vi "CASE Experiment Refinement.vi"() -> ()   [LabVIEW 2014]
uses:
  <vilib>/Simulation/Scripting/Companion Diagram/SimConfigNode/SimParams.ctl
  <vilib>/Simulation/Scripting/Companion Diagram/SimConfigNode/_simSolvers.ctl
  <vilib>/Simulation/Implementation/Shared/SIMSCR Execution Mode.ctl
  <vilib>/Platform/TimedLoop/XDataNode/timing_clust.ctl
  <vilib>/Platform/TimedLoop/XDataNode/nitl_modes.ctl
  <vilib>/Platform/TimedLoop/XDataNode/wakeup.ctl
  <vilib>/Simulation/Param Hierarchy/Typedefs/SIMPH Param Control Actions.ctl
  <vilib>/addons/control/pid/pid.llb/PID Structure.ctl
  <vilib>/addons/control/pid/pid.llb/PID Gain Unit.ctl
  <vilib>/Simulation/Implementation/Shared/NILVSim_ParamChanged.vi
  <vilib>/Simulation/Implementation/Shared/NILVSim_FinishedLate.vi
  <vilib>/Simulation/Implementation/Shared/NILVSIM_BeginStep.vi
  <vilib>/Simulation/ContinuousLinear/Implementation/NILVSim Transfer Function.llb/SIM Transfer Function Distributor (SISO).vi
  <vilib>/Simulation/ContinuousLinear/Implementation/NILVSim Transport Delay.llb/SIM Transport Delay Direct (scalar).vi
  <vilib>/Simulation/ContinuousLinear/Implementation/NILVSim Transfer Function.llb/SIM Transfer Function Collector (SISO).vi
  <vilib>/Simulation/SignalDisplay/Implementation/NILVSim Time Waveform.llb/SIM Time Waveform (vector).vi
  <vilib>/Simulation/Implementation/Shared/NILVSim_Manager.vi
  <vilib>/Utility/error.llb/Clear Errors.vi
  <vilib>/Simulation/Implementation/Shared/NILVSim_FinalizeModel.vi
  <vilib>/FPGAPlugInAG/myRIO-1900/niLvFpga_Open_myRIO-1900.vi
  <vilib>/rvi/interface/common/dynamic/niFpgaDynamicAddResources.vi
  <vilib>/Utility/error.llb/Error Cluster From Error Code.vi
  <vilib>/rvi/errors/niLvFpgaAdjustHostInterfaceError.vi
  <vilib>/Utility/file.llb/Write To Spreadsheet File (DBL).vi
  <vilib>/FPGAPlugInAG/Dynamic/niLvFpga_Close_Dynamic.vi
  <vilib>/Simulation/Implementation/Shared/SIM Unbundle Sim Info.vi
  <vilib>/Simulation/Implementation/Shared/SIMSH Read Queue.vi
  <vilib>/Simulation/Implementation/Shared/NILVSim_Initialize.vi
  <vilib>/addons/control/pid/pid.llb/PID Structure Conversion.vi
  <vilib>/addons/control/pid/pid.llb/PID Structure Conversion (DBL).vi
  <vilib>/addons/control/pid/pid.llb/PID Lead-Lag.vi
  <vilib>/addons/control/pid/pid.llb/PID Lead-Lag (DBL).vi
  <vilib>/addons/control/pid/pid.llb/PID Advanced.vi
  <vilib>/addons/control/pid/pid.llb/PID Advanced (DBL).vi
  <vilib>/Simulation/Utility/Implementation/NILVSim Get Time and IsAcceptedStep.vi
  <vilib>/Simulation/Implementation/Shared/NILVSim_GetModelError.vi
  <vilib>/Simulation/Implementation/Shared/SIM Bundle Sim Info.vi
  <vilib>/addons/Control Design/_Model Construction/Special Model Creation.llb/Special Model Creation SubVI/CD Create Pade Delay Model.vi
  <vilib>/addons/Control Design/_Model Construction/Special Model Creation.llb/Special Model Creation SubVI/CD Create 2nd Order Model.vi
  <vilib>/rvi/interface/nirviOpenFPGA/nirviOpenFPGA.xnode
  FPGA Bitfiles/Test_FPGATarget_CurrentControl_60eBuCSPTsI.lvbitx
  Current Control.vi
  <vilib>/rvi/interface/nirviReadWriteControl/nirviReadWriteControl.xnode
  <vilib>/rvi/interface/nirviCloseFPGA/nirviCloseFPGA.xnode
  <vilib>/Simulation/Scripting/Companion Diagram/SimConfigNode/SimDog.xnode
  <vilib>/Platform/TimedLoop/XDataNode/XDataNode.xnode
  <vilib>/Simulation/Implementation/XNodeFramework/SimXNode/SimX.xnode
  <vilib>/rvi/interface/Simulation/niFpgaSimulationCallBeginRW.vi
  <vilib>/addons/Control Design/_Model Construction/NI_LinSys_Model Creation.lvlib
  <vilib>/addons/Control Design/_Model Construction/Model Creation.llb/Model Creation SubVI/cd_Create Zero-Pole-Gain Model.vi
  <vilib>/addons/Control Design/_Model Conversions/NI_CD_Model Type.lvlib
  <vilib>/addons/Control Design/_Model Conversions/Model Type.llb/Model Conversion SubVI/cd_Convert Zero-Pole-Gain to Transfer Function Model.vi
  <vilib>/addons/Control Design/_Model Delay/NI_CD_Model Delay.lvlib
  <vilib>/addons/Control Design/_Model Delay/Model Delay.llb/Model Delay subVIs/cd_Convert Delay with Pade Approx (TF).vi
  <vilib>/addons/Control Design/_Model Interconnection/NI_CD_Model Interconnection.lvlib
  <vilib>/addons/Control Design/_Model Interconnection/Model Interconnection.llb/Model Interconnection SubVI/cd_Series (TF and TF).vi
  <vilib>/addons/control/pid/NI_PID_pid.lvlib
  <vilib>/addons/Control Design/_Model Construction/NI_CD_Special Model Creation.lvlib
  <vilib>/Simulation/ContinuousLinear/Implementation/NILVSim Transfer Function.llb/SIM Transfer Function (SISO).vi
  <vilib>/Utility/file.llb/Write To Spreadsheet File (I64).vi
  NiFpgaLv.dll
  <vilib>/Platform/TimedLoop/XDataNode/XDNodeRunTimeDep.lvlib
  <vilib>/Simulation/Implementation/Shared/NI_SIM_Implementation.lvlib
panel:
  out "PV1:":dbl(slide)=50.762476114859936 scale=0.0..100.0
  in  "ControlTab":enum32{"PID Parameters", "PI Parameters"}(tab)
  in  "PID BETA":dbl(slide)=1.0 scale=0.0..1.0
  in  "Gamma PID":dbl(slide) scale=0.0..1.0
  in  "Manual Mode PID":dbl(slide) scale=0.0..50.0
  in  "auto? (T)":bool=TRUE
  in  "reinitialize? (F)":bool
  in  "Linearity PID":dbl(slide)=1.0 scale=0.0..1.0
  in  "Alpha PID":dbl(slide)=nan scale=0.0..1.0
  in  "Feedforward\nLag Time (min)":dbl(slide)=0.9102981779915218 scale=0.01..10.0
  in  "auto? (T) PI":bool=TRUE
  in  "PI beta":dbl(slide)=1.0 scale=0.0..1.0
  in  "reinitialize? PI":bool
  in  "Linearity PI":dbl(slide)=1.0 scale=0.0..1.0
  in  "Alpha PI":dbl(slide)=nan scale=0.0..1.0
  in  "Gamma PI":dbl(slide)=nan scale=0.0..1.0
  in  "Manual Mode PI":dbl(slide) scale=0.0..50.0
  out "PI Gains":T1
  out "PD Gains":T1
  out "Error":errorcluster
  in  "?":enum32{"RT Response", "Excitation/Response"}(tab)
  in  "SP1:":dbl(slide)=40.87020302841148 min=0.0 max=0.0 scale=20.0..27.45
  out "MV1:":dbl(slide)=100.0 scale=-100.0..100.0
  out "SP2:":dbl(slide)=140.87020302841148 min=0.0 max=0.0 scale=0.0..100.0
  out "control valve":dbl=86.66603993277398 format="%.2f"
  out "Kinect Measurement vs. IAB Height":waveform(dbl)[](graph)
  out "Ref Head Pose":dbl(slide)=50.762476114859936 scale=20.0..27.0
  out "Bladder\nHeight":dbl(slide)=49.279730305904245 scale=0.0..100.0 scale format="%.2f"
  out "Process Chart":cluster{"SP1:":dbl, "output":dbl, "output":dbl}(graph)
  in  "stop":bool
  out "Status?":bool
  # "Instructions\n\nThis is a cascade PID and PI feedforward surge bladder controller\n\n1. Make sure the GAMMA value for the PID is set to 1 so as to apply the  max weight to the error value of the derivative kick action\n2. Make GAMMA for PI control action equal to 0 since we are not weighting the derivative kick here\n3. Linearity value should be 1 for both  controllers to avoid parabolic response. 1 makes your response linear.\n4. Alpha is the derivative filter time constant. To make the PID in feedforward critically damped, use a value of 1 here. Make Alpha for PI 0.\n5.  Beta is the value of the relative emphasis of disturbance rejection to setpoint tracking. Make Beta 1; else make beta between 0 and 1 to accommodate disturbances such as load changes\n\nCopyright June 2015. Olalekan P. Ogunmolu"
  # "Gamma specifies an amount by which to weight the error applied to derivative action. The default value is 0, which avoids the derivative kick, or sudden change in controller output, that can occur after a change in the setpoint value. Since this is a cascade PID, derivative kick is not a concern, increasing gamma might improve the speed of the first PID controller.\n\nBeta specifies the relative emphasis of disturbance rejection to setpoint tracking. The default value of 1 is appropriate for most applications. You can use a smaller value between 0 and 1 to specify emphasis on disturbance rejection, such as process load changes. This VI resizes the beta input array to match the size of the process variable input array. \n\nManual control specifies the value of the control output when auto? is FALSE. This VI resizes the manual control input array to match the size of the process variable input array. \n\nLinearity specifies the linearity of the error response. The valid range for linearity is 0 to 1. A value of 1 provides a normal linear response, while a value of 0.1 provides an approximately parabolic response. The VI uses this value in the nonlinear error calculation and the nonlinear gain factor calculation. \n\nAlpha specifies the derivative filter time constant. Increasing this value increases damping of derivative action. alpha can be a value between 0 and 1 or NaN, which specifies that no derivative filter is applied. \n\nAuto? specifies whether to use automatic or manual control. In some situations, you might need to switch off the PID controller and operate the system in manual, or open-loop, mode. The default is TRUE. When auto? is TRUE, this VI uses automatic control. When auto? is FALSE, this VI uses manual control. This VI uses bumpless transfer from manual control to automatic control."
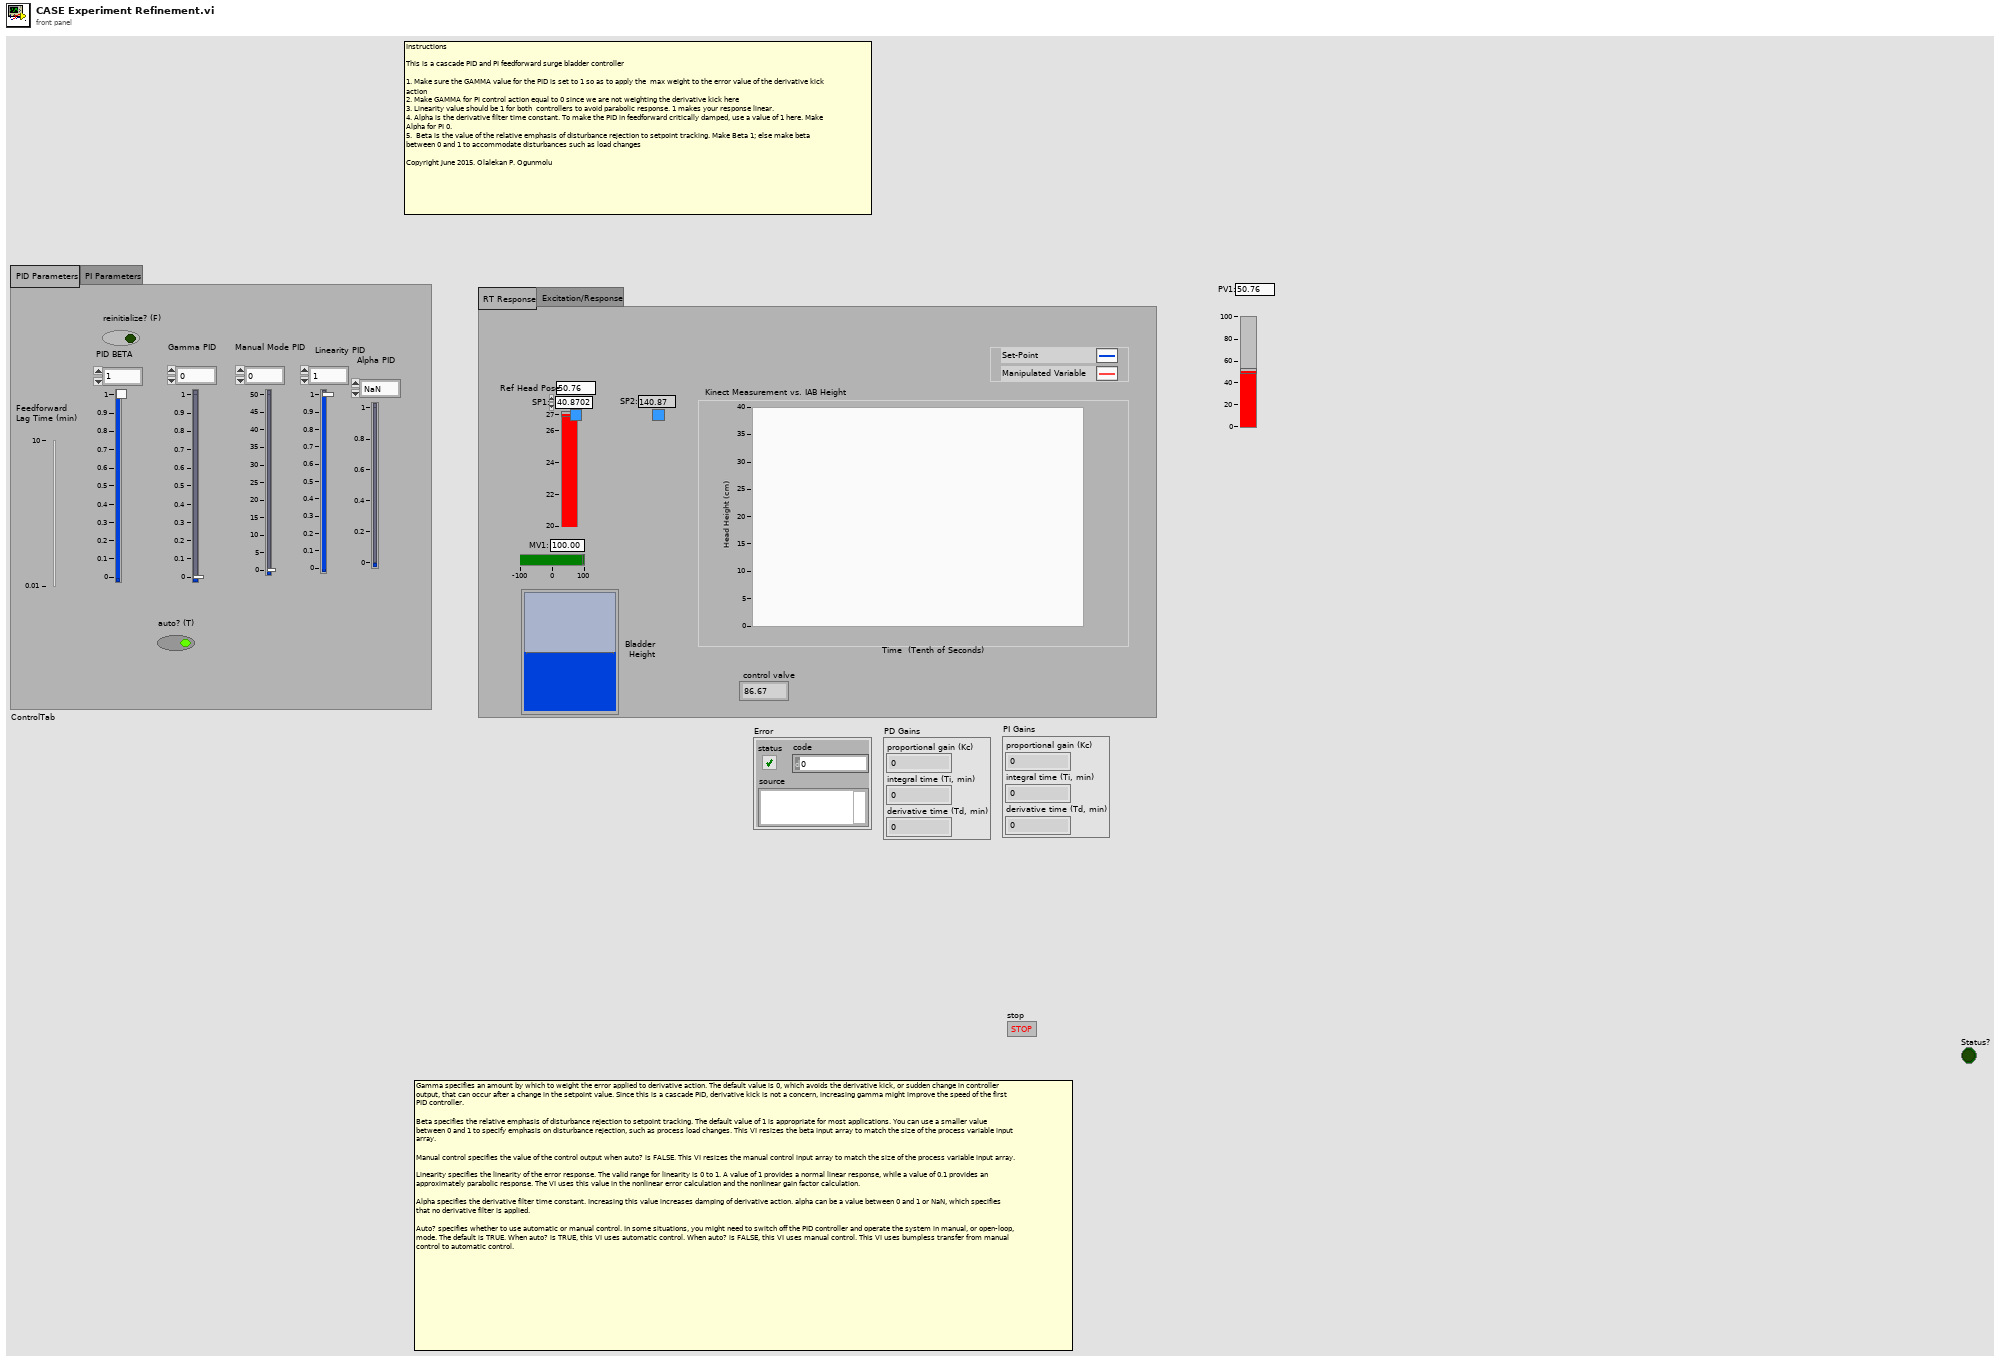
[diagram p1: front panel]
types:
  T1 = cluster{"proportional gain (Kc)":dbl, "integral time (Ti, min)":dbl, "derivative time (Td, min)":dbl}
  T2 = enum16{"big-endian, network order", "native, host order", "little-endian"}
  T3 = typedef "NI_LinSys_Model Typedefs.lvlib/CD Zero-Pole-Gain Model (MIMO).ctl" = cluster{"properties":T4, "zero-pole-gain(s)":T5[][]}
  T4 = typedef "NI_LinSys_Model Typedefs.lvlib/CD General Elements.ctl" = cluster{"Model name":string, "Input names":string[], "Output names":string[], "Input Delays":dbl[], "Output Delays":dbl[], "Sampling Time":dbl, "Notes":string}
  T5 = typedef "NI_LinSys_Model Typedefs.lvlib/CD Zero-Pole-Gain Model (SISO).ctl" = cluster{"Gain":dbl, "Zeros":cdb[], "Poles":cdb[], "delay":dbl}
  T6 = typedef "NI_LinSys_Model Typedefs.lvlib/CD Transfer Function Model (MIMO).ctl" = cluster{"properties":T4, "transfer function(s)":T7[][]}
  T7 = typedef "NI_LinSys_Model Typedefs.lvlib/CD Transfer Function Model (SISO).ctl" = cluster{"Numerator":dbl[], "Denominator":dbl[], "delay":dbl}
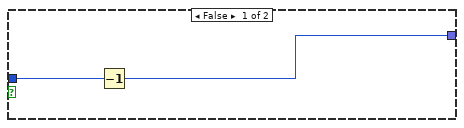
[diagram p4: hidden frame]
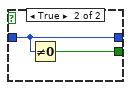
[diagram p5: hidden frame]
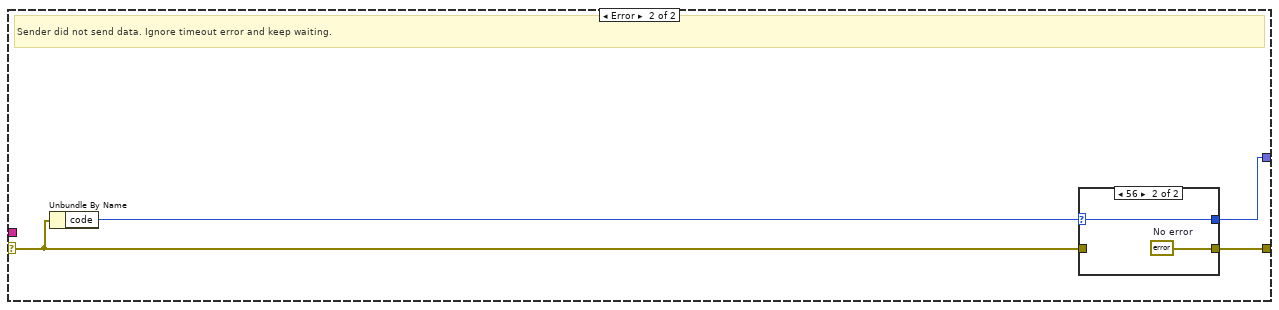
[diagram p6: hidden frame]
diagram:
  w14 = "192.168.1.5"  # address
  w13 = u16 80  # receiver port
  n1 = node-c288() -> (w5:variant)  [unwired: 1 in]
  n2 = node-c254 "Control & Simulation Loop"(w5) -> (w4:variant)
  n3 = String To IP(1:w14) -> (0:w15:u32)
  n4 = xnode "Open FPGA VI Reference"() -> ("FPGA VI Reference Out"=w7:refnum<k20>, "error out"=w6:errorcluster)  [unwired: 2 in]
  n5 = UDP Open(7:w15, 11:w13) -> (port=w12:refnum<k16>, 0:w11:errorcluster)  [unwired: 3 in, 1 out]
  n6 = while {
    tunnel: w12 -> [w43]
    tunnel: w11 -> [w42]
    tunnel: w7 -> [w37]
    tunnel: [w38] -> w9
    tunnel: w6 -> [w40]
    tunnel: [w39] -> w8
    tunnel: [w22] -> _
    tunnel: [w21] -> w10
    stop <- "stop" stop-if-true
    (unwired) u32 16777216
    # "Inflate Bladder to a max Current of 189mA from 60mA based on controller determination"
    n7 = Wait (ms)(milliseconds to wait=u32 50) -> ()  [unwired: 1 out]
    n8 = UDP Read(connection ID=w43, timeout ms (25000)=100, 8:w42) -> (data out=w24:string, error out=w23:errorcluster, 3:w21:refnum<k16>)  [unwired: 3 out]
    n9 = case shown="No Error" w23 {
      selector: w23 -> [w50 w87]
      tunnel: w24 -> [w51 _]
      tunnel: [w49 w86] -> w22
      tunnel: [w45 w85] -> _
      frame No Error {
        # "Loop"
        n10 = Unflatten From String(type=0, binary string=w51, data includes array or string size? (T)=FALSE, byte order (0:big-endian, network order)=T2."big-endian, network order" ("byte order"), error in (no error)=w50) -> (value=w52:i32, error out=w49:errorcluster)  [unwired: 1 out]
        n11 = To Long Integer(number=w52) -> (32bit integer=w47:i32)
        n12 = case shown="False" TRUE {
          tunnel: w47 -> [w81 w83]
          tunnel: [FALSE w84] -> w46
          tunnel: [w81 w83] -> w44
          frame False {
          }
          frame True {
            n13 = Not Equal To 0?(x=w83) -> (x != 0?=w84:bool)
          }
        }
        n14 = case shown="True" w46 {
          tunnel: w44 -> [w63 w79]
          tunnel: [w62 w77] -> w45
          frame False {
            n15 = Decrement(x=w63) -> (x-1=w62:i32)
          }
          frame True {
            n16 = local read "PV1:"() -> (w70:dbl)
            n17 = Subtract(x=w79, y=fxp<+,18,8> 246.3818359375) -> (x-y=w77:fxp<+/-,43,33>)
            n18 = Subtract(x=w70, y=0.0) -> (x-y=w69:dbl)
            n19 = Reciprocal(x=w69) -> (1/x=w68:dbl)
            n20 = Divide(x=w77, y=10.0) -> (x/y=w75:dbl)
            "PV1:" <- w75
            n21 = Multiply(x=w68, y=1000.0) -> (x*y=w66:dbl)
            n22 = Add(x=w66, y=2.0) -> (x+y=→"Ref Head Pose":dbl)
            n23 = Build Array(w75) -> (w76:dbl[])
            n24 = call-poly <vilib>:"Write To Spreadsheet File.vi"("format (%.3f)"="%.4f", "append to file? (new file:F)"=TRUE, "1D data"=w76, "file path (dialog if empty)"=path "c:/kinect2.csv") -> ()  [unwired: 4 in, 1 out]
          }
        }
        n25 = disable-structure shown="Disabled" {
          disable-tunnel: w45 -> [w56 _]
          frame Disabled {
            n26 = Build Array(w56) -> (w61:fxp<+/-,43,33>[])
            n27 = call-poly <vilib>:"Write To Spreadsheet File.vi"("delimiter (\\t)"="\\t" ("delimiter (\\t)"), "format (%d)"="%.2f", "append to file? (new file:F)"=TRUE, "1D data"=w61, "file path (dialog if empty)"=path "c:/kinectdata.csv") -> ()  [unwired: 3 in, 1 out]
          }
          frame Enabled {
          }
        }
      }
      frame Error {
        # "Sender did not send data. Ignore timeout error and keep waiting."
        n28 = Unbundle By Name(w87) -> ("code"=w88:i32)
        n29 = case shown="56" w88 {
          selector: w88 -> [w89 w91]
          tunnel: w87 -> [w90 _]
          tunnel: [w90 w92] -> w86
          tunnel: [w89 w91] -> w85
          frame Default {
          }
          frame 56 {
            w92 = errorcluster {"status"=FALSE, "code"=0, "source"=""}  # No error
          }
        }
      }
    }
    n30 = local read "Bladder\nHeight"() -> (w16:dbl)
    n31 = Multiply(x=w16, y=11.0) -> (x*y=w18:dbl)
    n32 = Multiply(x=w18, y=10200.0) -> (x*y=w25:dbl)
    n33 = Divide(x=w25, y=4.883) -> (x/y=w28:dbl)
    n34 = Multiply(x=w28, y=0.001) -> (x*y=w34:dbl)
    n35 = xnode "Read/Write Control"("FPGA VI Reference In"=w37, "error in"=w40, "DAC Inlet Valve"=w34) -> ("FPGA VI Reference Out"=w36:refnum<k20>, "error out"=w35:errorcluster)
    n36 = xnode "Read/Write Control"("FPGA VI Reference In"=w36, "error in"=w35) -> ("FPGA VI Reference Out"=w38:refnum<k20>, "error out"=w39:errorcluster, "Inlet Overflow?"=w33:bool)
    n37 = Unbundle By Name(w39) -> ("status"=w31:bool)
    n38 = Compound Arithmetic op=OR(w31, w33, FALSE ("value")) -> (→"Status?":bool)
  }
  n39 = disable-structure shown="Disabled" {
    frame Disabled {
      n40 = call-poly <vilib>:"CD Construct Zero-Pole-Gain Model.vi"("Gain"=0.0006, "Poles"=cdb[] [0.01+0.0i, 0.1028+0.0i], "Zeros"=cdb[] [1.7137+0.0i]) -> ("Zero-Pole-Gain Model"=w96:T3)  [unwired: 7 in, 1 out]
      n41 = call-poly <vilib>:"CD Convert to Transfer Function Model.vi"("Zero-Pole-Gain Model"=w96) -> ("Transfer Function Model"=w95:T6)  [unwired: 9 in, 1 out]
      n42 = call-poly <vilib>:"CD Series.vi"("Model 1"=w95) -> ()  [unwired: 9 in, 2 out]
      n43 = call-poly <vilib>:"CD Convert Delay with Pade Approximation.vi"() -> ("Transfer Function Converted Model"=w93:T6, "Transfer Function Model"=w94:T6)  [unwired: 9 in, 1 out]
    }
    frame Enabled {
    }
  }
  n44 = call-poly <vilib>:"CD Construct Special TF Model.vi"() -> ()  [unwired: 10 in, 2 out]
  n45 = call-poly <vilib>:"CD Construct Special TF Model.vi"() -> ()  [unwired: 10 in, 2 out]
  n46 = property on="ControlTab" class="TabCtl (strict)"("FG Color"=u32 16777226) -> ()  [unwired: 2 in, 2 out]
  n47 = property class="TabCtl (strict)"("FG Color"=u32 16777226) -> ()  [unwired: 2 in, 2 out]
  n48 = node-c288(w4) -> (→"Error":errorcluster)
  n49 = xnode "Close FPGA VI Reference"("FPGA VI Reference In"=w9, "error in"=w8) -> ()  [unwired: 1 out]
  n50 = UDP Close(connection ID=w10, 8:w8) -> ()  [unwired: 2 out]
